vi "Conditional Error to Warning.vi"(6 "Error Code":i32, 8 "error in":errorcluster) -> (0 "error out":errorcluster)   [LabVIEW 2009, in "POLARIS BME DG.lvlib"]
doc: "Resets error bit if error code matchs the in input \"Error Code\" specified.\n\n--------------\n\nauthor: Alexander Kessler, Helmholtz-Institut-Jena \nmaintainer: Alexander Kessler: alexander.kessler@uni-jena.de\n\nLicense Agreement for this software:\n\nCopyright (C)\nHelmholtz-Institut-Jena\nFröbelsteg 3\n07743 Jena\nGermany\n\nContact: alexander.kessler@uni-jena.de\n\nThis program is free software; you can redistribute it and/or modify it under the terms of the GNU General Public License as published by the Free Software Foundation; either version 2 of the license, or (at your option) any later version.\n\nThis program is distributed in the hope that it will be useful, but WITHOUT ANY WARRANTY; without even the implied warranty of MERCHANTABILITY or FITNESS FOR A PARTICULAR PURPOSE. See the GNU General License for more details (http://www.gnu.org)."
uses:
  POLARIS BME DG.lvlib
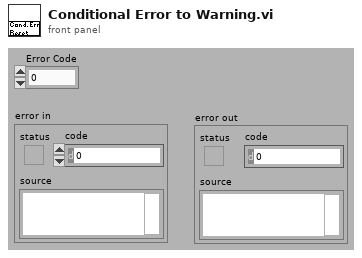
[diagram p1: front panel]
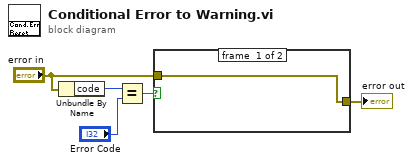
[diagram p0: block diagram]
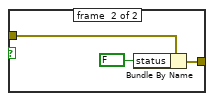
[diagram p2: hidden frame]
diagram:
  n1 = Unbundle By Name("error in") -> ("code"=w2:i32)
  n2 = Equal?(x=w2, y="Error Code") -> (x = y?=w1:bool)
  n3 = case shown="False" w1 {
    tunnel: [w6 w9] -> w5
    tunnel: "error in" -> [w6 w8]
    frame #0 {
    }
    frame #1 {
      n4 = Bundle By Name(cluster=w8, "status"=FALSE) -> (w9:errorcluster)
    }
  }
  "error out" <- w5
